vi "Expand Array To Size.vi"(5 "Default Value":dbl format="%.2f", 6 "Boolean Array In":bool[](array[boolean]), 7 "# Elements":i32, 8 "String Array In":string[](array[string]), 9 "2D U8 Array In":u8[][](array[numeric]), 10 "DBL Array In":dbl[](array[numeric]) format="%.2f", 11 "I32 Array In":i32[](array[numeric])) -> (0 "String Array Out":string[](array[string]), 1 "2D U8 Array Out":u8[][](array[numeric]), 2 "DBL Array Out":dbl[](array[numeric]) format="%.2f", 3 "I32 Array Out":i32[](array[numeric]), 4 "Boolean Array Out":bool[](array[boolean]))   [LabVIEW 2024]
panel:
  # "If input array has the specified number of elements or more, it is not changed.\nIf input array has less than specified number of elements, it is padded using the default value."
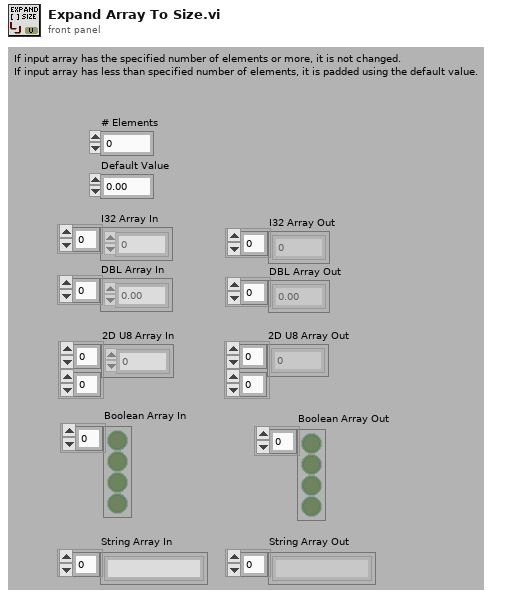
[diagram p1: front panel]
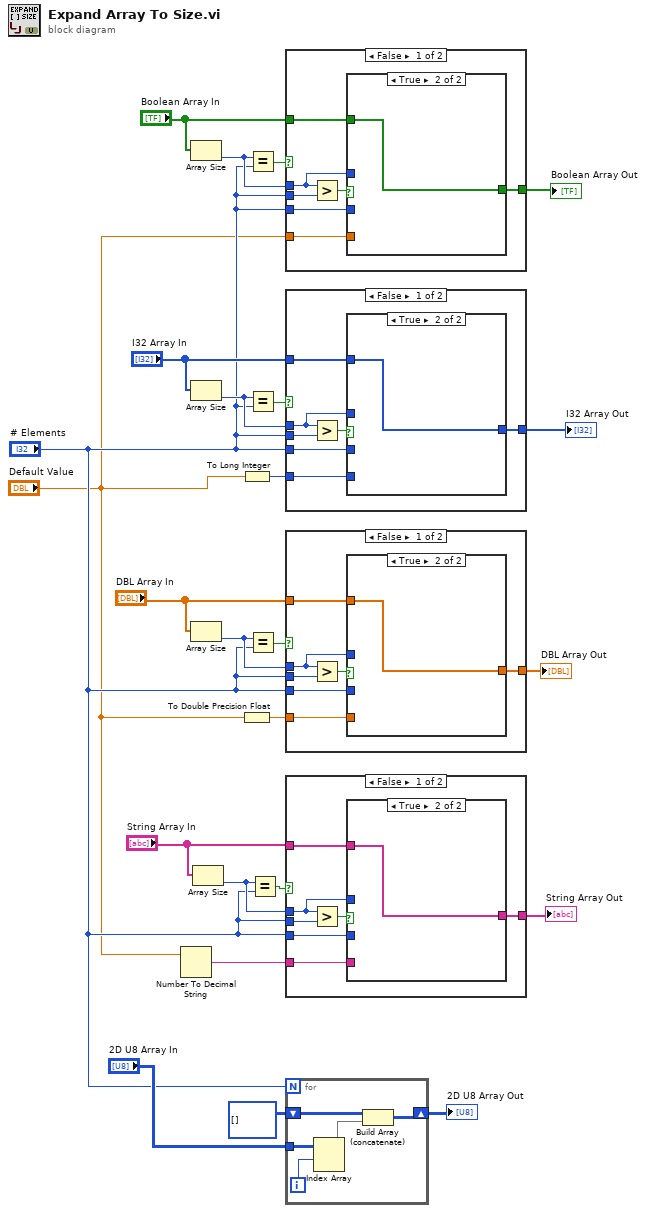
[diagram p0: block diagram]
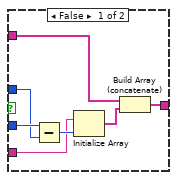
[diagram p2: hidden frame]
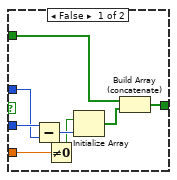
[diagram p4: hidden frame]
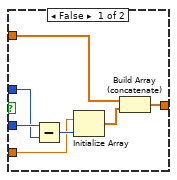
[diagram p6: hidden frame]
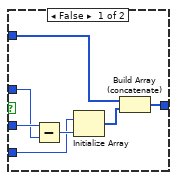
[diagram p8: hidden frame]
diagram:
  n1 = Number To Decimal String(number="Default Value") -> (decimal integer string=w2:string)  [unwired: 1 in]
  n2 = Array Size(array="Boolean Array In") -> (size(s)=w10:i32)
  n3 = Array Size(array="I32 Array In") -> (size(s)=w24:i32)
  n4 = Array Size(array="DBL Array In") -> (size(s)=w17:i32)
  n5 = Array Size(array="String Array In") -> (size(s)=w5:i32)
  n6 = To Long Integer(number="Default Value") -> (32bit integer=w21:i32)
  n7 = To Double Precision Float(number="Default Value") -> (double precision float=w19:dbl)
  n8 = Equal?(x=w10, y="# Elements") -> (x = y?=w11:bool)
  n9 = Equal?(x=w24, y="# Elements") -> (x = y?=w23:bool)
  n10 = Equal?(x=w17, y="# Elements") -> (x = y?=w18:bool)
  n11 = Equal?(x=w5, y="# Elements") -> (x = y?=w7:bool)
  n12 = case shown="False" w11 {
    tunnel: w10 -> [w26 _]
    tunnel: "# Elements" -> [w31 _]
    tunnel: "# Elements" -> [w29 _]
    tunnel: "Boolean Array In" -> [w28 w41]
    tunnel: [w27 w41] -> w8
    tunnel: "Default Value" -> [w25 _]
    frame False {
      n13 = Greater?(x=w26, y=w31) -> (0:w30:bool)
      n14 = case shown="True" w30 {
        tunnel: w29 -> [w39 _]
        tunnel: w28 -> [w35 w40]
        tunnel: [w34 w40] -> w27
        tunnel: w26 -> [w38 _]
        tunnel: w25 -> [w33 _]
        frame False {
          n15 = Subtract(x=w39, y=w38) -> (x-y=w37:i32)
          n16 = Not Equal To 0?(x=w33) -> (x != 0?=w32:bool)
          n17 = Initialize Array(w32, w37) -> (w36:bool[])
          n18 = Build Array (concatenate)(w35, w36) -> (w34:bool[])
        }
        frame True {
        }
      }
    }
    frame True {
    }
  }
  "Boolean Array Out" <- w8
  n19 = case shown="False" w23 {
    tunnel: w24 -> [w43 _]
    tunnel: "# Elements" -> [w48 _]
    tunnel: "# Elements" -> [w46 _]
    tunnel: "I32 Array In" -> [w45 w57]
    tunnel: [w44 w57] -> w20
    tunnel: w21 -> [w42 _]
    frame False {
      n20 = Greater?(x=w43, y=w48) -> (0:w47:bool)
      n21 = case shown="True" w47 {
        tunnel: w46 -> [w55 _]
        tunnel: w45 -> [w50 w56]
        tunnel: [w49 w56] -> w44
        tunnel: w43 -> [w54 _]
        tunnel: w42 -> [w52 _]
        frame False {
          n22 = Subtract(x=w55, y=w54) -> (x-y=w53:i32)
          n23 = Initialize Array(w52, w53) -> (w51:i32[])
          n24 = Build Array (concatenate)(w50, w51) -> (w49:i32[])
        }
        frame True {
        }
      }
    }
    frame True {
    }
  }
  "I32 Array Out" <- w20
  n25 = case shown="False" w18 {
    tunnel: w17 -> [w59 _]
    tunnel: "# Elements" -> [w64 _]
    tunnel: "# Elements" -> [w62 _]
    tunnel: "DBL Array In" -> [w61 w73]
    tunnel: [w60 w73] -> w16
    tunnel: w19 -> [w58 _]
    frame False {
      n26 = Greater?(x=w59, y=w64) -> (0:w63:bool)
      n27 = case shown="True" w63 {
        tunnel: w62 -> [w71 _]
        tunnel: w61 -> [w66 w72]
        tunnel: [w65 w72] -> w60
        tunnel: w59 -> [w70 _]
        tunnel: w58 -> [w68 _]
        frame False {
          n28 = Subtract(x=w71, y=w70) -> (x-y=w69:i32)
          n29 = Initialize Array(w68, w69) -> (w67:dbl[])
          n30 = Build Array (concatenate)(w66, w67) -> (w65:dbl[])
        }
        frame True {
        }
      }
    }
    frame True {
    }
  }
  "DBL Array Out" <- w16
  n31 = case shown="False" w7 {
    tunnel: w5 -> [w75 _]
    tunnel: "# Elements" -> [w80 _]
    tunnel: "# Elements" -> [w78 _]
    tunnel: "String Array In" -> [w77 w89]
    tunnel: [w76 w89] -> w1
    tunnel: w2 -> [w74 _]
    frame False {
      n32 = Greater?(x=w75, y=w80) -> (0:w79:bool)
      n33 = case shown="True" w79 {
        tunnel: w78 -> [w87 _]
        tunnel: w77 -> [w82 w88]
        tunnel: [w81 w88] -> w76
        tunnel: w75 -> [w86 _]
        tunnel: w74 -> [w84 _]
        frame False {
          n34 = Subtract(x=w87, y=w86) -> (x-y=w85:i32)
          n35 = Initialize Array(w84, w85) -> (w83:string[])
          n36 = Build Array (concatenate)(w82, w83) -> (w81:string[])
        }
        frame True {
        }
      }
    }
    frame True {
    }
  }
  "String Array Out" <- w1
  n37 = for {
    N: "# Elements" -> [_]
    shift-right: [w90] -> w13
    shift-left: u8[][] [] -> [w91]
    tunnel: "2D U8 Array In" -> [w94]
    i -> [w93]
    n38 = Index Array(array=w94, index (row)=w93) -> (element=w92:u8[])  [unwired: 1 in]
    n39 = Build Array (concatenate)(w91, w92) -> (w90:u8[][])
  }
  "2D U8 Array Out" <- w13
